vi "g_ImageCalibration.vi"() -> ()   [LabVIEW 2014]
panel:
  out "Factor Pix -> mm":dbl
  out "Factor Pix -> um":dbl
  in  "Micrometer Reference":dbl=2769.16
  in  "Pixel Reference":dbl=364.0
  # "References based on Calibration within Vision Builder\nUpdate when Camera or other settings change"
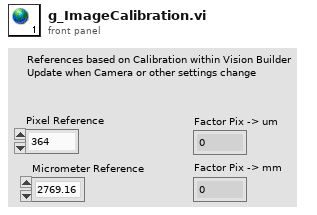
[diagram p1: front panel]
diagram:
